vi "Read Line.vi"(8 "error in":errorcluster, 10 "Previous":string, 11 "VISA resource name":refnum<visa-resource-name>) -> (0 "error out":errorcluster, 1 "Length":u32, 2 "Message":string, 3 "VISA resource name out":refnum<visa-resource-name>, 4 "Remaining":string)   [LabVIEW 2019, in "Andeen-Hagerling 2700.lvlib"]
doc: "Read a line from the selected VISA resource. Line terminates at the line feed character."
uses:
  Andeen-Hagerling 2700.lvlib
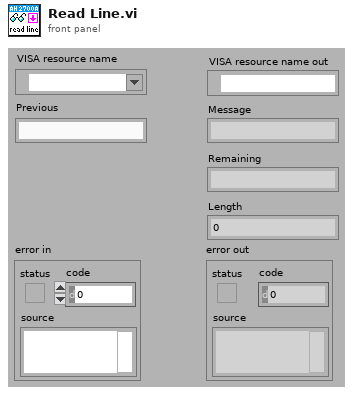
[diagram p1: front panel]
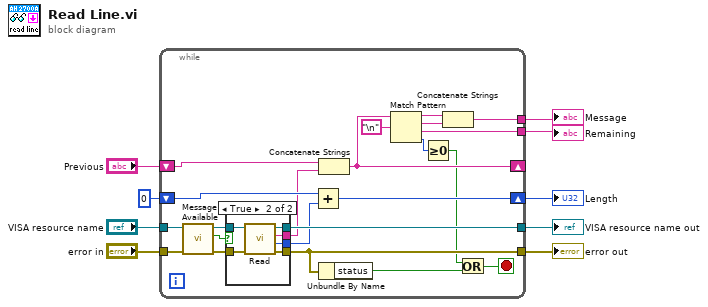
[diagram p0: block diagram]
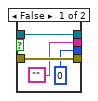
[diagram p2: hidden frame]
diagram:
  n1 = while {
    tunnel: "error in" -> [w31]
    tunnel: "VISA resource name" -> [w30]
    tunnel: [w25] -> w6
    tunnel: [w26] -> w5
    shift-right: [w23] -> w4
    shift-left: u32 0 -> [w22]
    shift-right: [w19] -> _
    shift-left: "Previous" -> [w20]
    tunnel: [w11] -> w2
    tunnel: [w10] -> w3
    stop <- w14 stop-if-true
    n2 = call "Message Available.vi"("error in"=w31, "VISA resource name"=w30) -> ("error out"=w27:errorcluster, "message available"=w29:bool, "VISA resource name out"=w28:refnum<visa-resource-name>)  [unwired: 7 in]
    n3 = case shown="True" w29 {
      tunnel: w28 -> [w35 w41]
      tunnel: w27 -> [w34 w40]
      tunnel: [u32 0 ("Length") w39] -> w24
      tunnel: ["" w38] -> w21
      tunnel: [w35 w37] -> w26
      tunnel: [w34 w36] -> w25
      frame False {
      }
      frame True {
        n4 = call "Read.vi"("error in"=w40, "VISA resource name"=w41) -> ("error out"=w36:errorcluster, "Length"=w39:u32, "Message"=w38:string, "VISA resource name out"=w37:refnum<visa-resource-name>)  [unwired: 6 in]
      }
    }
    n5 = Add(x=w22, y=w24) -> (x+y=w23:u32)
    n6 = Concatenate Strings(w20, w21) -> (w19:string)
    n7 = Unbundle By Name(w25) -> ("status"=w15:bool)
    n8 = Match Pattern(string=w19, regular expression="\n") -> (before substring=w13:string, match substring=w12:string, after substring=w11:string, offset past match=w17:i32)  [unwired: 1 in]
    n9 = Greater Or Equal To 0?(x=w17) -> (x >= 0?=w16:bool)
    n10 = Concatenate Strings(w13, w12) -> (w10:string)
    n11 = Or(x=w16, y=w15) -> (x .or. y?=w14:bool)
  }
  "VISA resource name out" <- w5
  "error out" <- w6
  "Message" <- w3
  "Length" <- w4
  "Remaining" <- w2
